vi "2-input NOR.vi"(10 "Obtained Expression":string, 11 "Input List":string[](array[string])) -> (1 "O/p = I/p":string, 2 "Nand ?":bool, 3 "Logic Exp":string)   [LabVIEW 2014]
doc: "This VI is used to compare the obtained logic with the logic of NAND gate."
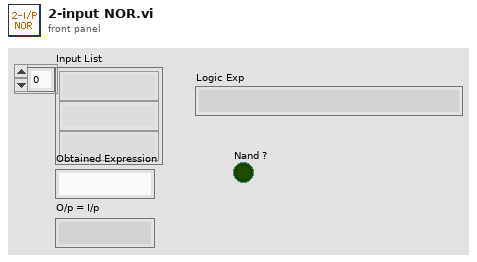
[diagram p1: front panel]
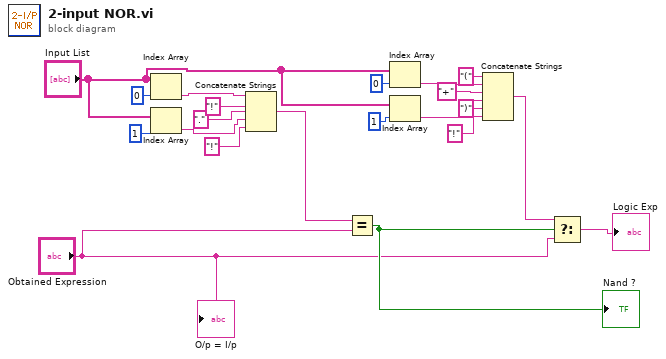
[diagram p0: block diagram]
diagram:
  n1 = Index Array(array="Input List", index=0) -> (element=w19:string)
  n2 = Index Array(array="Input List", index=1) -> (element=w21:string)
  n3 = Concatenate Strings(w19, "!" ("t"), "." ("string"), w21, "!" ("t")) -> (w5:string)
  n4 = Equal?(x=w5, y="Obtained Expression") -> (x = y?=w16:bool)
  "Nand ?" <- w16
  n5 = Index Array(array="Input List", index=0) -> (element=w12:string)
  n6 = Index Array(array="Input List", index=1) -> (element=w10:string)
  n7 = Concatenate Strings("(" ("string"), w12, "+" ("string"), w10, ")" ("string"), "!" ("string")) -> (w9:string)
  n8 = Select(t=w9, s=w16, f="Obtained Expression") -> (s? t:f=→"Logic Exp":string)
  "O/p = I/p" <- "Obtained Expression"
